vi "Analog data2waveform.vi"(11 "Queue in":refnum<queue>) -> (1 "last element":dbl, 2 "# elements in queue":i32, 3 "Waveform":cluster{"value":dbl, dbl, "elements":dbl[]})   [LabVIEW 2014]
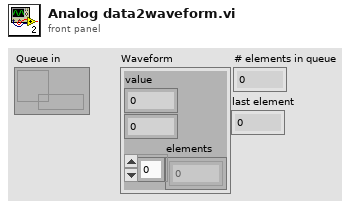
[diagram p1: front panel]
types:
  T1 = cluster{"start value":dbl, dbl, "elements":dbl[]}
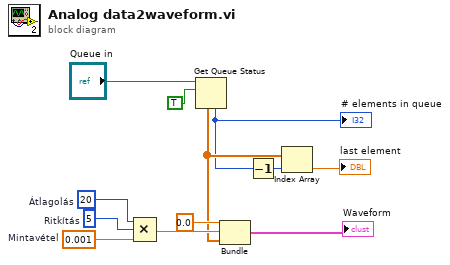
[diagram p0: block diagram]
diagram:
  w12 = 5  # Ritkítás
  w11 = 20  # Átlagolás
  w10 = 0.001  # Mintavétel
  n1 = Compound Arithmetic op=MULTIPLY(w11, w12, w10) -> (w5:dbl)
  n2 = Get Queue Status(queue="Queue in", return elements? (F)=TRUE) -> (# elements in queue=w2:i32, elements=w3:dbl[])  [unwired: 1 in, 6 out]
  "# elements in queue" <- w2
  n3 = Bundle("start value"=0.0, w5, "elements"=w3) -> (→"Waveform":T1)  [unwired: 1 in]
  n4 = Decrement(x=w2) -> (x-1=w4:i32)
  n5 = Index Array(array=w3, index=w4) -> (element=→"last element":dbl)
